vi "get_multiramp_soak_configuration.vi"(8 "error in (no error)":errorcluster, 10 "Configuration":string(combo)="0", 11 "VISA Refnum in":refnum<visa-resource-name>) -> (0 "error out":errorcluster, 3 "VISA Refnum out":refnum<visa-resource-name>)   [LabVIEW 2018]
panel:
  out "Configuration":string
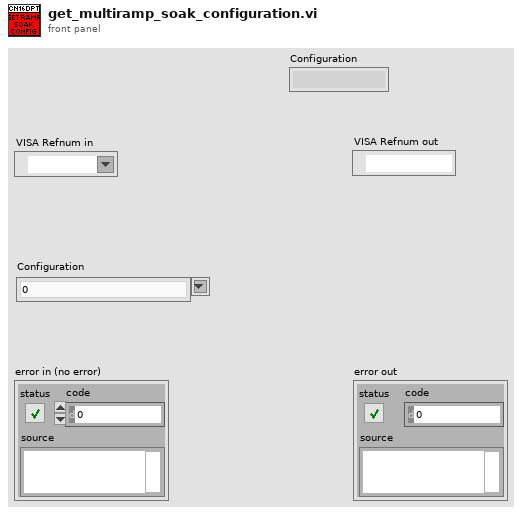
[diagram p1: front panel]
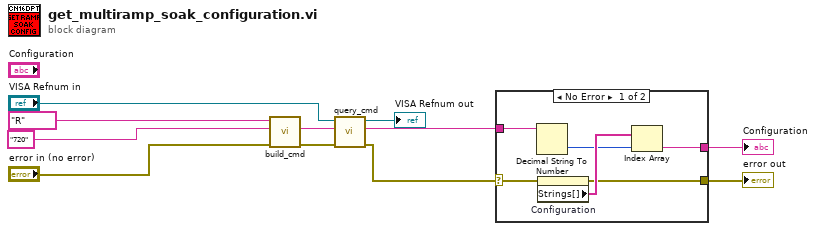
[diagram p0: block diagram]
diagram:
  n1 = call "build_cmd.vi"("error in (no error)"="error in (no error)", "Command ID"="720", "Command class"="R") -> ("error out"=w6:errorcluster, "Command"=w5:string)  [unwired: 7 in]
  n2 = call "query_cmd.vi"("error in (no error)"=w6, "Command"=w5, "VISA resource name"="VISA Refnum in") -> ("error out"=w3:errorcluster, "Response"=w4:string, "VISA resource name out"=→"VISA Refnum out":refnum<visa-resource-name>)  [unwired: 6 in]
  n3 = case shown="No Error" w3 {
    selector: w3 -> [w17 w18]
    tunnel: w4 -> [w16 _]
    tunnel: [w13 _] -> w1
    tunnel: [w12 w18] -> w2
    frame No Error {
      n4 = Decimal String To Number(string=w16) -> (number=w14:i32)  [unwired: 2 in, 1 out]
      n5 = property on="Configuration" class="CmbBox"(error in=w17) -> (error out=w12:errorcluster, "Strings[]"=w15:string[])  [unwired: 1 in, 1 out]
      n6 = Index Array(array=w15, index=w14) -> (element=w13:string)
    }
    frame Error {
    }
  }
  "error out" <- w2
  "Configuration" <- w1
